vi "create reporting folder path.vi"(8 "error in (no error)":errorcluster, 11 "Autofocus in":refnum<class "Autofocus.lvclass">) -> (0 "error out":errorcluster, 1 "full file path":path, 2 "folder base":path, 3 "Autofocus out":refnum<class "Autofocus.lvclass">)   [LabVIEW 2012, in "Autofocus.lvclass"]
uses:
  Autofocus.lvclass
  Autofocus.lvclass/Autofocus.ctl
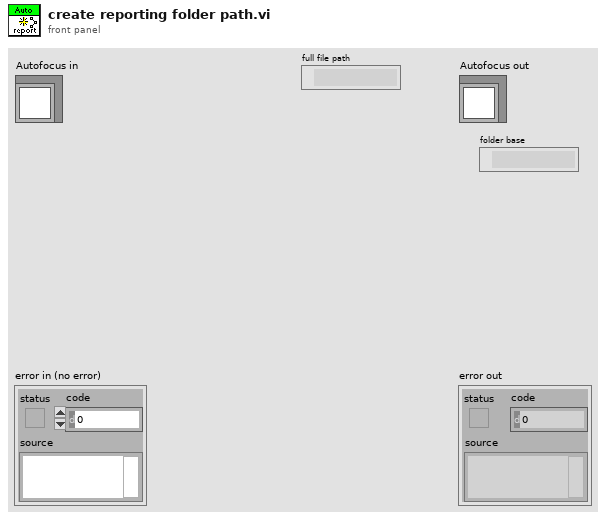
[diagram p1: front panel]
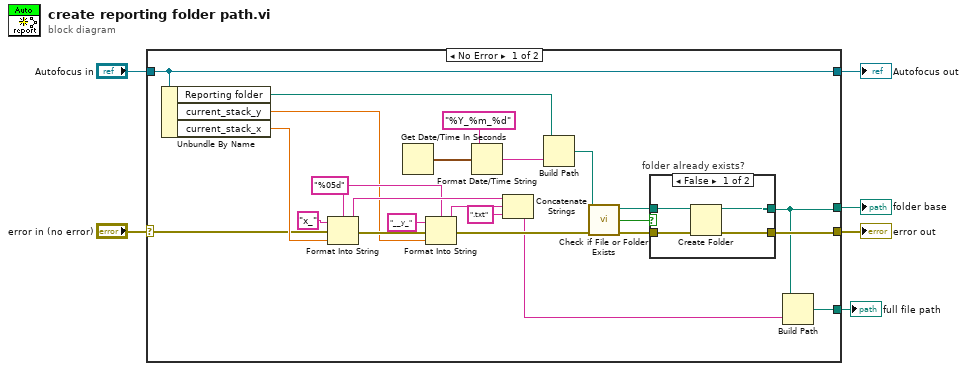
[diagram p0: block diagram]
diagram:
  n1 = case shown="No Error" "error in (no error)" {
    selector: "error in (no error)" -> [w20 w38]
    tunnel: [w10 w38] -> w5
    tunnel: [w30 w37] -> w3
    tunnel: "Autofocus in" -> [w30 w37]
    tunnel: [w9 _] -> w2
    tunnel: [w7 _] -> w1
    frame No Error {
      w26 = "%05d" ("format string")
      n2 = Unbundle By Name(w30) -> ("Reporting folder"=w16:path, "current_stack_y"=w21:dbl[unit], "current_stack_x"=w22:dbl[unit])
      n3 = Format Into String(format string=w26, initial string="x_", error in=w20, w22) -> (resulting string=w27:string, error out=w23:errorcluster)
      n4 = Get Date/Time In Seconds() -> (seconds since 1Jan1904=w17:timestamp)
      n5 = Format Into String(format string=w26, initial string="__y_", error in=w23, w21) -> (resulting string=w28:string, error out=w12:errorcluster)
      n6 = Format Date/Time String(time format string (%c)="%Y_%m_%d", seconds (now)=w17) -> (date/time string=w19:string)  [unwired: 1 in]
      n7 = Concatenate Strings(w27, w28, ".txt" ("string")) -> (w8:string)
      n8 = Build Path(base path=w16, name or relative path=w19) -> (appended path=w11:path)
      n9 = call <vilib>:"Check if File or Folder Exists.vi"("error in (no error)"=w12, "path"=w11) -> ("error out"=w14:errorcluster, "file or folder exists?"=w13:bool, "dup path"=w15:path)  [unwired: 7 in]
      n10 = case "folder already exists?" shown="False" w13 {
        tunnel: [w32 w36] -> w10
        tunnel: w14 -> [w34 w36]
        tunnel: w15 -> [w33 w35]
        tunnel: [w31 w35] -> w9
        frame False {
          n11 = Create Folder(path (use dialog)=w33, error in=w34) -> (created path=w31:path, error out=w32:errorcluster)  [unwired: 1 in, 1 out]
        }
        frame True {
        }
      }
      n12 = Build Path(base path=w9, name or relative path=w8) -> (appended path=w7:path)
    }
    frame Error {
    }
  }
  "error out" <- w5
  "Autofocus out" <- w3
  "folder base" <- w2
  "full file path" <- w1
